vi "winForms setPythonColor.vi"(2 "error in (no error)":errorcluster, 3 "stylesRefNum":refnum<k24>) -> (0 "error out":errorcluster)   [LabVIEW 2018]
uses:
  C:/ATI_MS_InstrumentControl/dll/ScintillaNET.dll
  dll/ScintillaNET.dll
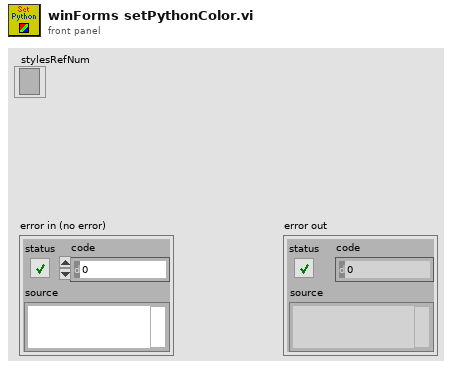
[diagram p1: front panel]
types:
  T1 = cluster{"style":i32, "color":u32, "bold":bool, "italic":bool, "fillLine":bool}
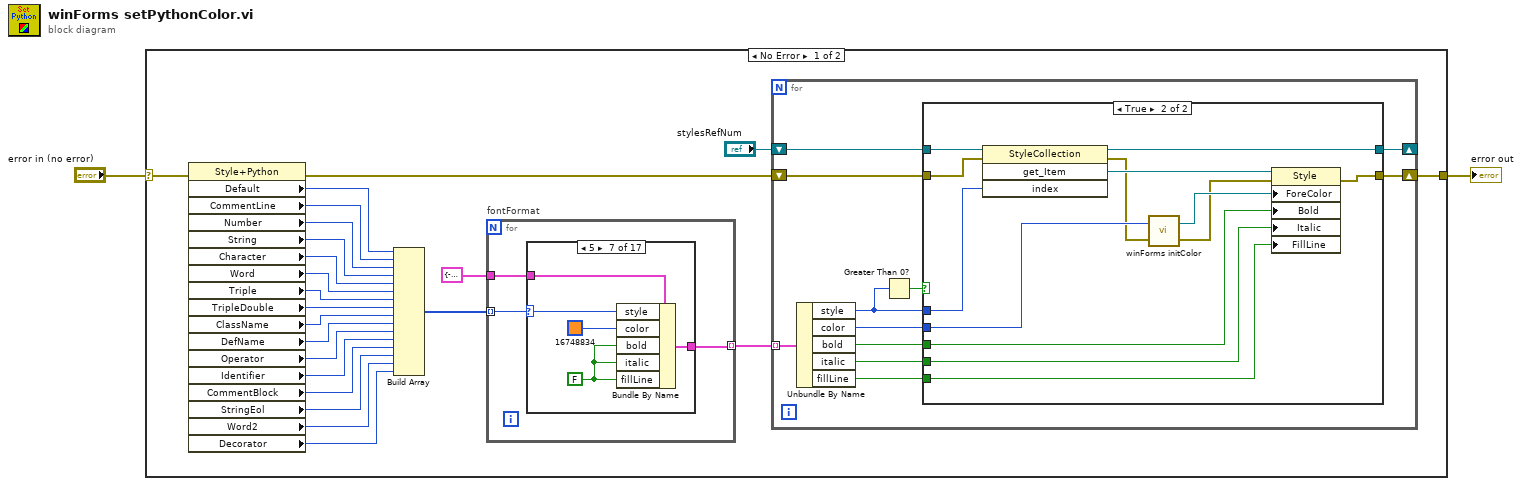
[diagram p0: block diagram]
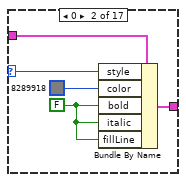
[diagram p4: hidden frame]
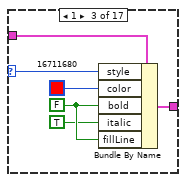
[diagram p5: hidden frame]
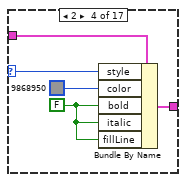
[diagram p6: hidden frame]
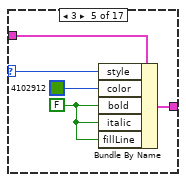
[diagram p7: hidden frame]
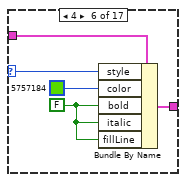
[diagram p8: hidden frame]
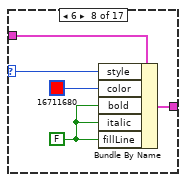
[diagram p9: hidden frame]
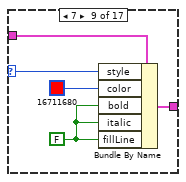
[diagram p10: hidden frame]
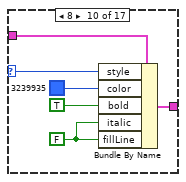
[diagram p11: hidden frame]
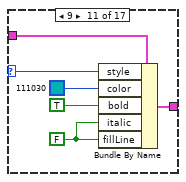
[diagram p12: hidden frame]
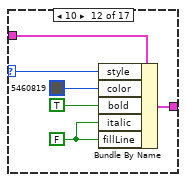
[diagram p13: hidden frame]
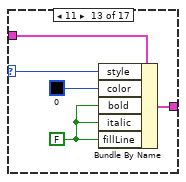
[diagram p14: hidden frame]
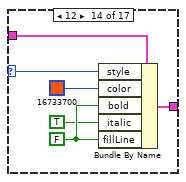
[diagram p15: hidden frame]
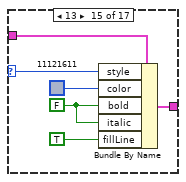
[diagram p16: hidden frame]
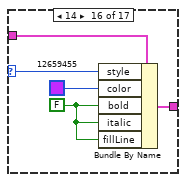
[diagram p17: hidden frame]
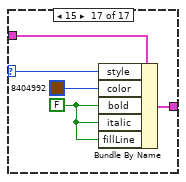
[diagram p18: hidden frame]
diagram:
  n1 = case shown="No Error" "error in (no error)" {
    selector: "error in (no error)" -> [w3 w142]
    tunnel: [w4 w142] -> w2
    frame No Error {
      n2 = property class="Style+Python"(error in=w3) -> (error out=w5:errorcluster, "Default"=w25:i32, "CommentLine"=w24:i32, "Number"=w23:i32, "String"=w22:i32, "Character"=w21:i32, "Word"=w20:i32, "Triple"=w19:i32, "TripleDouble"=w18:i32, "ClassName"=w17:i32, "DefName"=w16:i32, "Operator"=w15:i32, "Identifier"=w14:i32, "CommentBlock"=w13:i32, "StringEol"=w12:i32, "Word2"=w11:i32, "Decorator"=w10:i32)  [unwired: 1 in, 1 out]
      n3 = Build Array(w25, w24, w23, w22, w21, w20, w19, w18, w17, w16, w15, w14, w13, w12, w11, w10) -> (w6:i32[])
      n4 = for "fontFormat" {
        tunnel: T1 {"style"=-1, "color"=0, "bold"=FALSE, "italic"=FALSE, "fillLine"=FALSE} -> [w54]
        tunnel: [w53] -> w8 mode=indexing
        tunnel: w6 -> [w52] mode=indexing
        n5 = case shown="5" w52 {
          selector: w52 -> [_ w56 w61 w67 w72 w77 w83 w87 w92 w97 w103 w109 w115 w120 w126 w132 w137]
          tunnel: w54 -> [w55 w60 w66 w71 w76 w81 w86 w91 w96 w102 w108 w114 w119 w125 w131 w136 w141]
          tunnel: [w55 w57 w63 w69 w74 w79 w84 w89 w94 w100 w106 w112 w117 w123 w129 w135 w140] -> w53
          frame -1, Default {
          }
          frame 0 {
            w58 = FALSE ("bold")
            n6 = Bundle By Name(cluster=w60, "style"=w56, "color"=u32 8289918, "bold"=w58, "italic"=w58, "fillLine"=w58) -> (w57:T1)
          }
          frame 1 {
            w64 = FALSE ("bold")
            n7 = Bundle By Name(cluster=w66, "style"=w61, "color"=u32 16711680, "bold"=w64, "italic"=TRUE, "fillLine"=w64) -> (w63:T1)
          }
          frame 2 {
            w68 = FALSE ("bold")
            n8 = Bundle By Name(cluster=w71, "style"=w67, "color"=u32 9868950, "bold"=w68, "italic"=w68, "fillLine"=w68) -> (w69:T1)
          }
          frame 3 {
            w73 = FALSE ("bold")
            n9 = Bundle By Name(cluster=w76, "style"=w72, "color"=u32 4102912, "bold"=w73, "italic"=w73, "fillLine"=w73) -> (w74:T1)
          }
          frame 4 {
            w78 = FALSE ("bold")
            n10 = Bundle By Name(cluster=w81, "style"=w77, "color"=u32 5757184, "bold"=w78, "italic"=w78, "fillLine"=w78) -> (w79:T1)
          }
          frame 5 {
            w82 = FALSE ("bold")
            n11 = Bundle By Name(cluster=w86, "style"=w83, "color"=u32 16748834, "bold"=w82, "italic"=w82, "fillLine"=w82) -> (w84:T1)
          }
          frame 6 {
            w88 = FALSE ("bold")
            n12 = Bundle By Name(cluster=w91, "style"=w87, "color"=u32 16711680, "bold"=w88, "italic"=w88, "fillLine"=w88) -> (w89:T1)
          }
          frame 7 {
            w93 = FALSE ("bold")
            n13 = Bundle By Name(cluster=w96, "style"=w92, "color"=u32 16711680, "bold"=w93, "italic"=w93, "fillLine"=w93) -> (w94:T1)
          }
          frame 8 {
            w99 = FALSE ("bold")
            n14 = Bundle By Name(cluster=w102, "style"=w97, "color"=u32 3239935, "bold"=TRUE, "italic"=w99, "fillLine"=w99) -> (w100:T1)
          }
          frame 9 {
            w105 = FALSE ("bold")
            n15 = Bundle By Name(cluster=w108, "style"=w103, "color"=u32 111030, "bold"=TRUE, "italic"=w105, "fillLine"=w105) -> (w106:T1)
          }
          frame 10 {
            w111 = FALSE ("bold")
            n16 = Bundle By Name(cluster=w114, "style"=w109, "color"=u32 5460819, "bold"=TRUE, "italic"=w111, "fillLine"=w111) -> (w112:T1)
          }
          frame 11 {
            w116 = FALSE ("bold")
            n17 = Bundle By Name(cluster=w119, "style"=w115, "color"=u32 0, "bold"=w116, "italic"=w116, "fillLine"=w116) -> (w117:T1)
          }
          frame 12 {
            w122 = FALSE ("bold")
            n18 = Bundle By Name(cluster=w125, "style"=w120, "color"=u32 16733700, "bold"=w122, "italic"=TRUE, "fillLine"=w122) -> (w123:T1)
          }
          frame 13 {
            w128 = FALSE ("bold")
            n19 = Bundle By Name(cluster=w131, "style"=w126, "color"=u32 11121611, "bold"=w128, "italic"=w128, "fillLine"=TRUE ("bold")) -> (w129:T1)
          }
          frame 14 {
            w133 = FALSE ("bold")
            n20 = Bundle By Name(cluster=w136, "style"=w132, "color"=u32 12659455, "bold"=w133, "italic"=w133, "fillLine"=w133) -> (w135:T1)
          }
          frame 15 {
            w138 = FALSE ("bold")
            n21 = Bundle By Name(cluster=w141, "style"=w137, "color"=u32 8404992, "bold"=w138, "italic"=w138, "fillLine"=w138) -> (w140:T1)
          }
        }
      }
      n22 = for {
        tunnel: w8 -> [w36] mode=indexing
        shift-right: [w30] -> _
        shift-left: "stylesRefNum" -> [w31]
        shift-right: [w28] -> w4
        shift-left: w5 -> [w29]
        n23 = Unbundle By Name(w36) -> ("style"=w27:i32, "color"=w35:u32, "bold"=w34:bool, "italic"=w33:bool, "fillLine"=w32:bool)
        n24 = Greater Than 0?(x=w27) -> (x > 0?=w26:bool)
        n25 = case shown="True" w26 {
          tunnel: w35 -> [_ w51]
          tunnel: w34 -> [_ w50]
          tunnel: w33 -> [_ w49]
          tunnel: w32 -> [_ w48]
          tunnel: w31 -> [w38 w47]
          tunnel: [w38 w46] -> w30
          tunnel: w29 -> [w37 w45]
          tunnel: [w37 w44] -> w28
          tunnel: w27 -> [_ w39]
          frame False {
          }
          frame True {
            n26 = invoke class="StyleCollection" method="get_Item"(reference=w47, error in=w45, "index"=w39) -> (reference out=w46:refnum<k24>, error out=w42:errorcluster, "get_Item"=w43:refnum<k24>)  [unwired: 1 in, 1 out]
            n27 = call "winForms initColor.vi"("error in (no error)"=w42, "Color Box"=w51) -> ("error out"=w40:errorcluster, "reference out"=w41:refnum<k24>)
            n28 = property class="Style"(reference=w43, error in=w40, "ForeColor"=w41, "Bold"=w50, "Italic"=w49, "FillLine"=w48) -> (error out=w44:errorcluster)  [unwired: 1 out]
          }
        }
      }
    }
    frame Error {
    }
  }
  "error out" <- w2
